vi "Map Channel Info to VS SDI Channels.vi"(9 "label":i32, 10 "Tx Channels Array":string[](array[string]), 11 "Rx Channels Array":string[](array[string])) -> (2 "Tx Channels Array out":string[](array[string]), 3 "Rx Channels Array out":string[](array[string]))   [LabVIEW 2020, in "Single Board Loopback.lvclass"]
uses:
  Single Board Loopback.lvclass
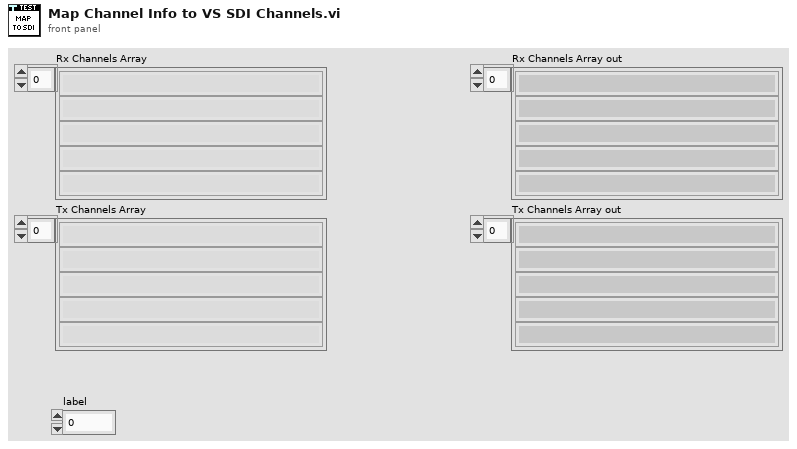
[diagram p1: front panel]
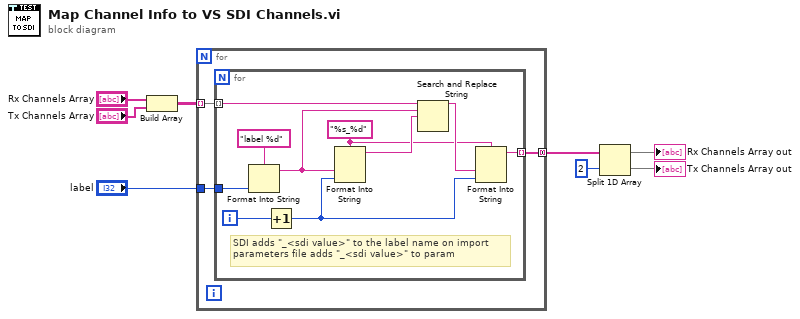
[diagram p0: block diagram]
diagram:
  n1 = Build Array("Rx Channels Array", "Tx Channels Array") -> (w5:string[][])
  n2 = for {
    tunnel: "label" -> [w11]
    tunnel: w5 -> [w10] mode=indexing
    tunnel: [w9] -> w4 mode=concatenating
    n3 = for {
      tunnel: w11 -> [w19]
      tunnel: w10 -> [w21] mode=indexing
      tunnel: [w15] -> w9 mode=indexing
      i -> [w13]
      w12 = "%s_%d" ("format string")
      # "SDI adds \"_<sdi value>\" to the label name on import\nparameters file adds \"_<sdi value>\" to param"
      n4 = Format Into String(format string="label %d", w19) -> (resulting string=w18:string)  [unwired: 2 in, 1 out]
      n5 = Increment(x=w13) -> (x+1=w14:i32)
      n6 = Format Into String(format string=w12, w18, w14) -> (resulting string=w17:string)  [unwired: 2 in, 1 out]
      n7 = Search and Replace String(input string=w21, search string=w18, replace string=w17) -> (result string=w16:string)  [unwired: 5 in, 3 out]
      n8 = Format Into String(format string=w12, w16, w14) -> (resulting string=w15:string)  [unwired: 2 in, 1 out]
    }
  }
  n9 = Split 1D Array(array=w4, index=2 ("dimension size")) -> (first subarray=→"Rx Channels Array out":string[], second subarray=→"Tx Channels Array out":string[])
